vi "Panel.vi"(11 "GaugeEditorPanel in":refnum<class "GaugeEditorPanel.lvclass">) -> ()   [LabVIEW 2020, in "VolatusGUIControls.lvlib" / "GaugeEditorPanel.lvclass"]
uses:
  GaugeEditorPanel.lvclass
panel:
  # "No custom editor is available for this control."
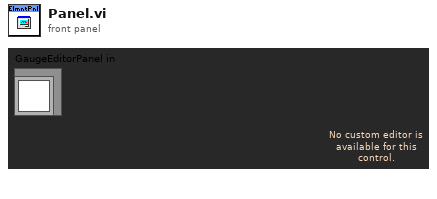
[diagram p1: front panel]
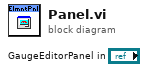
[diagram p0: block diagram]
diagram:
